vi "Specific Error Handler.vi"   [LabVIEW 2017]
doc: "Checks an error against a set of error handling instructions configured by the express VI.\n\nIf the error to check is in the list of errors to handle, the VI extracts the error handling information and performs the apropriate actions.\n\nThis VI will never detect an error with a code of 0, even if the status is set to true."
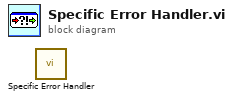
[diagram p0: block diagram]
diagram:
  n1 = call "Specific Error Handler"() -> ()  [unwired: 12 in, 4 out]
